vi "Example 1.vi"() -> ()   [LabVIEW 2020]
uses:
  FINS/FINS_header.ctl
  FINS/FINS CMD.ctl
  subvi/task.ctl
  FINS/FINS TCP.lvlib
panel:
  out "x-y":u32
  in  "address":u16=146
  out "Waveform Chart":sgl(graph)
  in  "stop":bool
  out "error o":errorcluster
  out "Numeric":sgl format="%.1f"
  out "data":bool[][](array[boolean])
  out "data":u8[](array[numeric])
  out "RSP":bool
  out "server Header":T1={"resp req"=FALSE, "cmd resp"=FALSE, "SID"=255, "DNA"=2, "DA1"=2, "DA2"=2, "SA1"=0, "SA2"=255, "SNA"=255} {"SNA" max=127 format="%x"; "SA2" max=254 step=1 format="%x"; "SA1" format="%x"; "DA2" max=254 step=1 format="%x"; "DA1" format="%x"; "DNA" max=127 step=1 format="%x"}
  out "server CMD":T2
  out "FINS Header":T1 {"SNA" max=127 format="%x"; "SA2" max=254 step=1 format="%x"; "SA1" format="%x"; "DA2" max=254 step=1 format="%x"; "DA1" format="%x"; "DNA" max=127 step=1 format="%x"}
  in  "SA1":u8 format="%x"
  out "Client Node":u32=10 format="%x"
  out "Server Node":u32=10 format="%x"
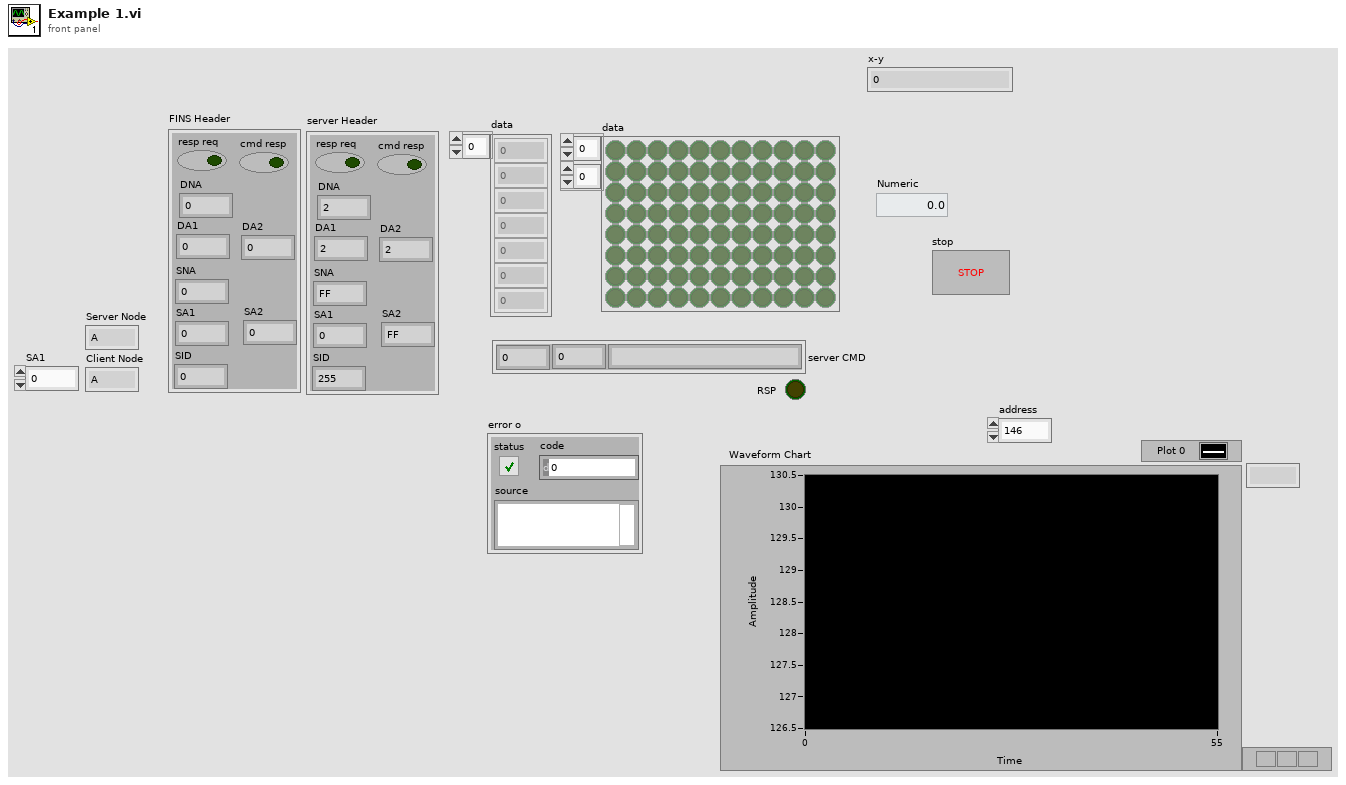
[diagram p1: front panel]
types:
  T1 = typedef "FINS TCP.lvlib/FINS_header.ctl" = cluster{"resp req":bool, "cmd resp":bool, "SID":u8, "DNA":u8, "DA1":u8, "DA2":u8, "SA1":u8, "SA2":u8, "SNA":u8}
  T2 = typedef "FINS TCP.lvlib/FINS CMD.ctl" = cluster{"MR":u8, "SR":u8, "name":string}
  T3 = typedef "task.ctl" = enum16{"connect", "send", "send-recv", "receive", "disconnect"}
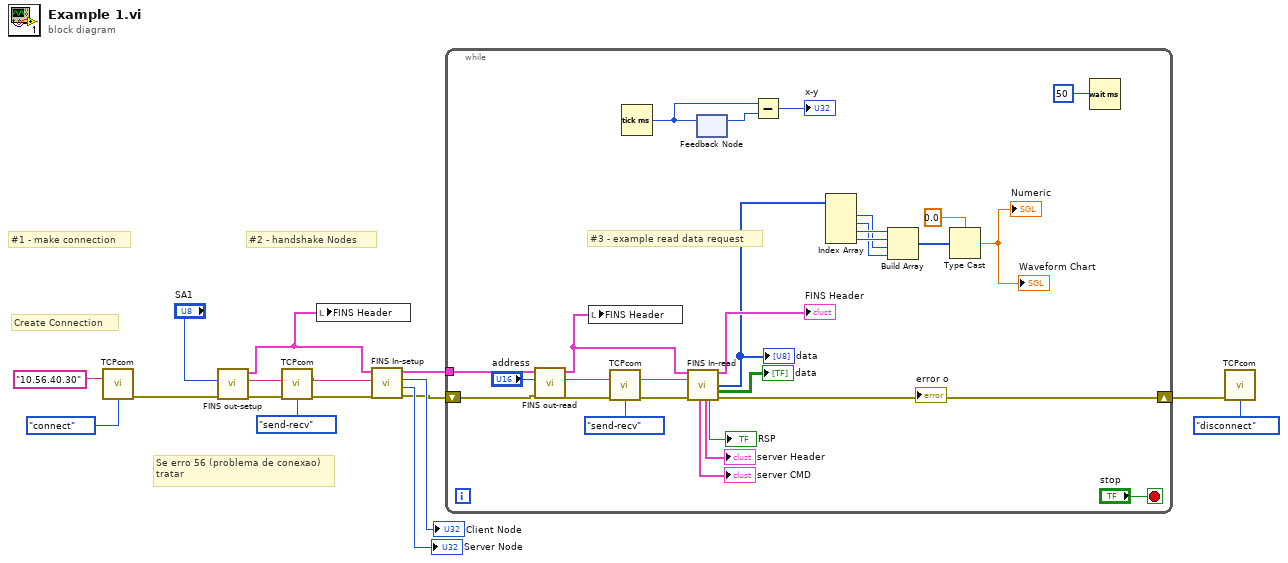
[diagram p0: block diagram]
diagram:
  # "Se erro 56 (problema de conexao)\ntratar"
  # "#2 - handshake Nodes"
  # "#1 - make connection"
  # "Create Connection"
  n1 = call "TCPcom.vi"("string"="10.56.40.30" ("address"), "task"=task."connect") -> ("error out"=w15:errorcluster)  [unwired: 12 in, 1 out]
  n2 = call "FINS out-setup.vi"("error i"=w15, "SA1"="SA1") -> ("error o"=w13:errorcluster, "msg"=w14:string, "FINS Header"=w3:T1)  [unwired: 7 in]
  n3 = call "TCPcom.vi"("string"=w14, "error in"=w13, "task"=task."send-recv") -> ("data out"=w11:string, "error out"=w10:errorcluster)  [unwired: 11 in]
  n4 = local write "FINS Header"(w3) -> ()
  n5 = call "FINS In-setup.vi"("error i"=w10, "msg 3"=w11, "FINS Header i"=w3) -> ("error o"=w4:errorcluster, "Server Node"=→"Server Node":u32, "Client Node"=→"Client Node":u32, "FINS Header o"=w5:T1)  [unwired: 5 in]
  n6 = while {
    tunnel: w5 -> [w43]
    shift-right: [w34] -> w1
    shift-left: w4 -> [w42]
    stop <- "stop" stop-if-true
    # "#3 - example read data request"
    n7 = call "FINS out-read.vi"("error i"=w42, "address"="address", "FINS Header 2"=w43) -> ("error o"=w40:errorcluster, "msg"=w41:string, "FINS Header"=w32:T1)  [unwired: 6 in]
    n8 = local write "FINS Header"(w32) -> ()
    n9 = call "TCPcom.vi"("string"=w41, "error in"=w40, "task"=task."send-recv") -> ("data out"=w39:string, "error out"=w38:errorcluster)  [unwired: 11 in]
    n10 = Tick Count (ms)() -> (millisecond timer value=w18:u32)
    n11 = call "FINS In-read.vi"("FINS Header i"=w32, "msg 3"=w39, "error i"=w38) -> ("FINS Header o"=→"FINS Header":T1, 8:"data"=w20:u8[], 10:"data"=→"data":bool[][], "CMD"=→"server CMD":T2, "FINS Header 2"=→"server Header":T1, "RSP"=→"RSP":bool, "error o"=w34:errorcluster)  [unwired: 6 in]
    "data" <- w20
    "error o" <- w34
    n12 = feedback-in #1(w18) -> ()
    n13 = feedback #1() -> (w19:u32)  [unwired: 1 in]
    n14 = Subtract(x=w18, y=w19) -> (x-y=→"x-y":u32)
    n15 = Index Array(array=w20) -> (element #1=w24:u8, element #2=w23:u8, element #3=w26:u8, element #4=w25:u8)  [unwired: 4 in]
    n16 = Build Array(w26, w25, w24, w23) -> (w22:u8[])
    n17 = Type Cast(type=sgl 0.0 ("Numeric"), x=w22) -> (*(type *) &x=→"Numeric" →"Waveform Chart":sgl)
    n18 = Wait (ms)(milliseconds to wait=u32 50 ("millisecond multiple")) -> ()  [unwired: 1 out]
  }
  n19 = call "TCPcom.vi"("error in"=w1, "task"=task."disconnect") -> ()  [unwired: 12 in, 2 out]
